vi "Add Current Sensors.vi"(11 "Sensors Info IN":T1(array[cluster]) {"Max Error % of Reading" format="%.2f"; "Max Stability Error" format="%.2f"; "Max Mean Squared Error" format="%.2f"; "Max Error % of Full Scale" format="%.2f"; "Coefficients" format="%.2f"; "Voltage List" format="%.2f"; "EGU List" format="%.2f"; "EGU Range"."Low Limit" format="%.2f"; "EGU Range"."High Limit" format="%.2f"; "Voltage Range"."Low Limit" format="%.2f"; "Voltage Range"."High Limit" format="%.2f"; "Last Cal Info"."Last Calibration Date" format="%.2f"}) -> (3 "Sensors Info OUT":T1(array[cluster]))   [LabVIEW 2019]
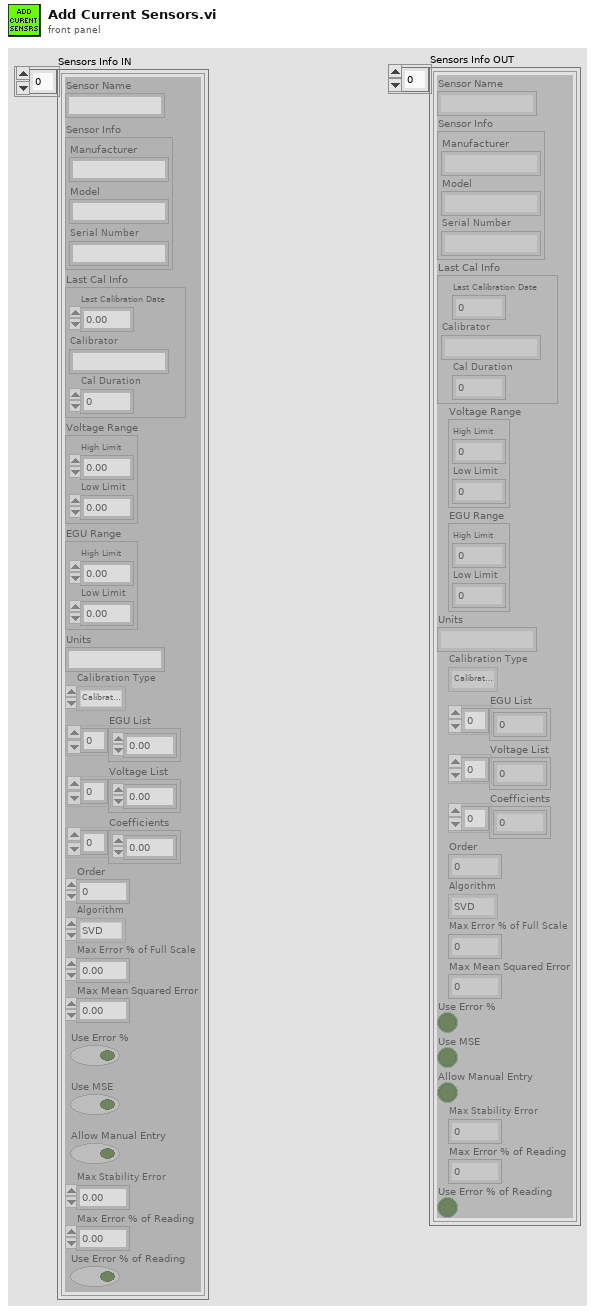
[diagram p1: front panel]
types:
  T1 = cluster{"Sensor Name":string, "Sensor Info":cluster{"Manufacturer":string, "Model":string, "Serial Number":string}, "Last Cal Info":cluster{"Last Calibration Date":dbl, "Calibrator":string, "Cal Duration":i32}, "Voltage Range":cluster{"High Limit":dbl, "Low Limit":dbl}, "EGU Range":cluster{"High Limit":dbl, "Low Limit":dbl}, "Units":string, "Calibration Type":enum16{"Calibrate Analog", "Compare Analog Calibration"}, "EGU List":dbl[], "Voltage List":dbl[], "Coefficients":dbl[], "Order":i32, "Algorithm":enum32{"SVD", "Givens", "Givens2", "Householder", "LU Decomposition", "Cholesky"}, "Max Error % of Full Scale":dbl, "Max Mean Squared Error":dbl, "Use Error %":bool, "Use MSE":bool, "Allow Manual Entry":bool, "Max Stability Error":dbl, "Max Error % of Reading":dbl, "Use Error % of Reading":bool}[]
  T2 = cluster{"Sensor Name":string, "Sensor Info":cluster{"Manufacturer":string, "Model":string, "Serial Number":string}, "Last Cal Info":cluster{"Last Calibration Date":dbl, "Calibrator":string, "Cal Duration":i32}, "Voltage Range":cluster{"High Limit":dbl, "Low Limit":dbl}, "EGU Range":cluster{"High Limit":dbl, "Low Limit":dbl}, "Units":string, "Calibration Type":enum16{"Calibrate Analog", "Compare Analog Calibration"}, "EGU List":dbl[], "Voltage List":dbl[], "Coefficients":dbl[], "Order":i32, "Algorithm":enum32{"SVD", "Givens", "Givens2", "Householder", "LU Decomposition", "Cholesky"}, "Max Error % of Full Scale":dbl, "Max Mean Squared Error":dbl, "Use Error %":bool, "Use MSE":bool, "Allow Manual Entry":bool, "Max Stability Error":dbl, "Max Error % of Reading":dbl, "Use Error % of Reading":bool}
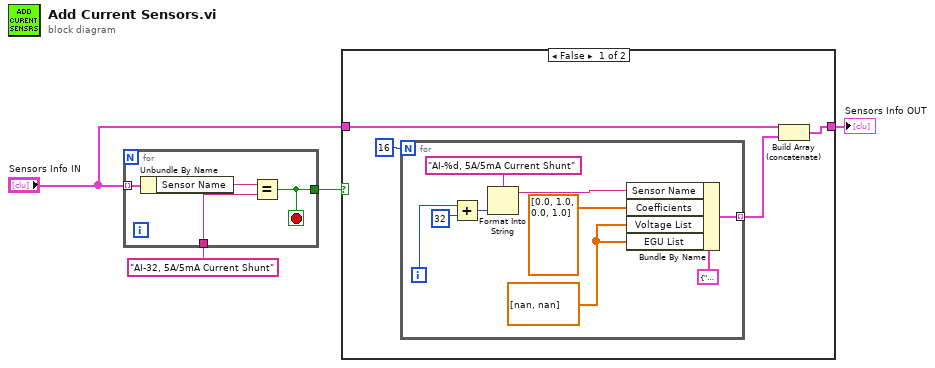
[diagram p0: block diagram]
diagram:
  n1 = for {
    tunnel: "Sensors Info IN" -> [w8] mode=indexing
    tunnel: [w6] -> w4
    tunnel: "AI-32, 5A/5mA Current Shunt" ("y") -> [w5]
    stop <- w6 stop-if-true
    n2 = Unbundle By Name(w8) -> ("Sensor Name"=w7:string)
    n3 = Equal?(x=w7, y=w5) -> (x = y?=w6:bool)
  }
  n4 = case shown="False" w4 {
    tunnel: "Sensors Info IN" -> [w11 w22]
    tunnel: [w10 w22] -> w2
    frame False {
      n5 = for {
        N: 16 -> [_]
        tunnel: [w13] -> w9 mode=indexing
        i -> [w21]
        w14 = dbl[] [nan, nan] ("Voltage List")
        n6 = Add(x=w21, y=32) -> (x+y=w19:i32)
        n7 = Format Into String(format string="AI-%d, 5A/5mA Current Shunt" ("y"), w19) -> (resulting string=w16:string)  [unwired: 2 in, 1 out]
        n8 = Bundle By Name(cluster=T2 {"Sensor Name"="", "Sensor Info"={"Manufacturer"="", "Model"="", "Serial Number"=""}, "Last Cal Info"={"Last Calibration Date"=0.0, "Calibrator"="", "Cal Duration"=0}, "Voltage Range"={"High Limit"=0.0, "Low Limit"=0.0}, "EGU Range"={"High Limit"=0.0, "Low Limit"=0.0}, "Units"="", "Calibration Type"=enum."Calibrate Analog", "EGU List"=[], "Voltage List"=[], "Coefficients"=[], "Order"=0, "Algorithm"=enum."SVD", "Max Error % of Full Scale"=0.0, "Max Mean Squared Error"=0.0, "Use Error %"=FALSE, "Use MSE"=FALSE, "Allow Manual Entry"=FALSE, "Max Stability Error"=0.0, "Max Error % of Reading"=0.0, "Use Error % of Reading"=FALSE} ("Sensor Description"), "Sensor Name"=w16, "Coefficients"=dbl[] [0.0, 1.0, 0.0, 1.0], "Voltage List"=w14, "EGU List"=w14) -> (w13:T2)
      }
      n9 = Build Array (concatenate)(w11, w9) -> (w10:T1)
    }
    frame True {
    }
  }
  "Sensors Info OUT" <- w2
